vi "Read Msg Header ID.vi"(8 "error in (no error)":errorcluster, 11 "RDS Message in":refnum<class "RDS Message.lvclass">) -> (0 "error out":errorcluster, 1 "Time Stamp":timestamp, 2 "Msg ID":T1, 3 "RDS Message out":refnum<class "RDS Message.lvclass">, 5 "Sender Name":string)   [LabVIEW 2015, in "RDS Child Messages.lvlib" / "RDS Message.lvclass"]
uses:
  RDS Message.lvclass
  RDS Message ID.ctl
  RDS Message.lvclass/RDS Message.ctl
  RDS Child Messages/RDS Child Messages.lvlib
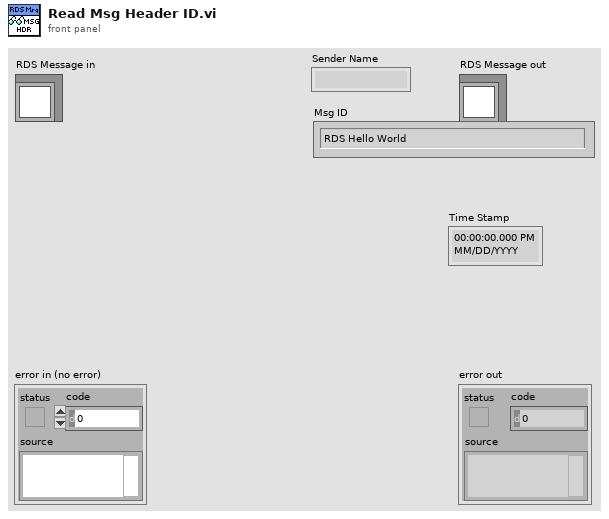
[diagram p1: front panel]
types:
  T1 = typedef "RDS Child Messages.lvlib/RDS Message ID.ctl" = enum16{"RDS Hello World", "String Message", "AIP_Status", "AIP_Command", "GPS_Data", "MCB_Command", "MCB_Status", "Compass_Data", "Depth_Data", "Battery_Data", "Contoller_State", "Set_Mag_Dev", "BTB_Shutdown", "State_Sample_Request", "State_Sample", "PID_Gains_Set", "Helm_Limiter_Set", "Helm_Heading_Command", "Helm_Steering_Command", "Helm_Status", "Controller_Message", "AIP_Set_Min_Depth", "Mission_Controller_State", "Mission_Upload", "Mission_Set_Op_and_Run", "Mission_Settings_Set"}
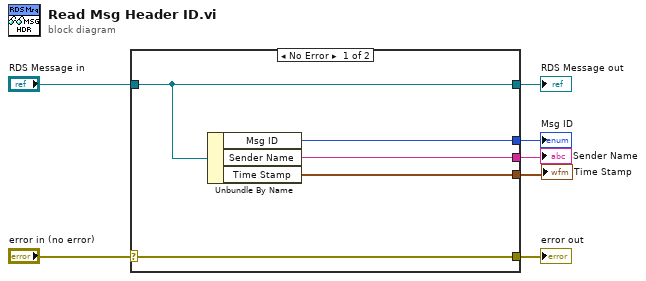
[diagram p0: block diagram]
diagram:
  n1 = case shown="No Error" "error in (no error)" {
    selector: "error in (no error)" -> [w12 w13]
    tunnel: [w12 w13] -> w6
    tunnel: [w11 w14] -> w4
    tunnel: "RDS Message in" -> [w11 w14]
    tunnel: [w10 _] -> w1
    tunnel: [w9 _] -> w3
    tunnel: [w8 _] -> w2
    frame No Error {
      n2 = Unbundle By Name(w11) -> ("Msg ID"=w10:T1, "Sender Name"=w9:string, "Time Stamp"=w8:timestamp)
    }
    frame Error {
    }
  }
  "error out" <- w6
  "RDS Message out" <- w4
  "Sender Name" <- w3
  "Time Stamp" <- w2
  "Msg ID" <- w1
